vi "Buscador de calor.vi"() -> ()   [LabVIEW 2010]
uses:
  <vilib>/Platform/TimedLoop/XDataNode/XDataNode.xnode
  <vilib>/Platform/TimedLoop/XDataNode/timing_clust.ctl
  <vilib>/Platform/TimedLoop/XDataNode/nitl_modes.ctl
  <vilib>/Platform/TimedLoop/XDataNode/wakeup.ctl
  <vilib>/Instr/_visa.llb/VISA Configure Serial Port (Instr).vi
  <vilib>/Platform/TimedLoop/XDataNode/XDNodeRunTimeDep.lvlib
panel:
  out "Lumenes":dbl(slide) scale=0.0..255.0
  out "String":string
  in  "Ajuste":dbl(slide) scale=0.1..1.0
  in  "Set Lumenes":dbl(slide) scale=50.0..255.0
  in  "Automatico/Manual":bool
  out "Temperatura (ºC) vs tiempo":dynamicdata(graph)
  in  "Intensidad Luminica (%)":dbl(knob) scale=10.0..100.0
  in  "Period                :":i64=1000
  in  "Flow control    :":u16(ring) items=["None"=0, "XON/XOFF"=1, "RTS/CTS"=2, "DTR/DSR"=4]
  in  "Stop bits         :":u16(ring)=10 items=["1.0"=10, "1.5"=15, "2.0"=20]
  in  "Paridad            :":u16(ring) items=["None", "Odd", "Even", "Mark", "Space"]
  in  "Data bits          :":u16=8 min=5 max=8 step=1
  in  "VISA resource : name:":refnum<visa-resource-name>="COM1"
  in  "Baud rate         :":u32=9600
  in  "stop":bool
  out "Read buffer":string
  out "var t":u8
  out "Auto 2":bool
  # "CONTROL INTENSIDAD LUMINICA"
  # "Configuracion Serial"
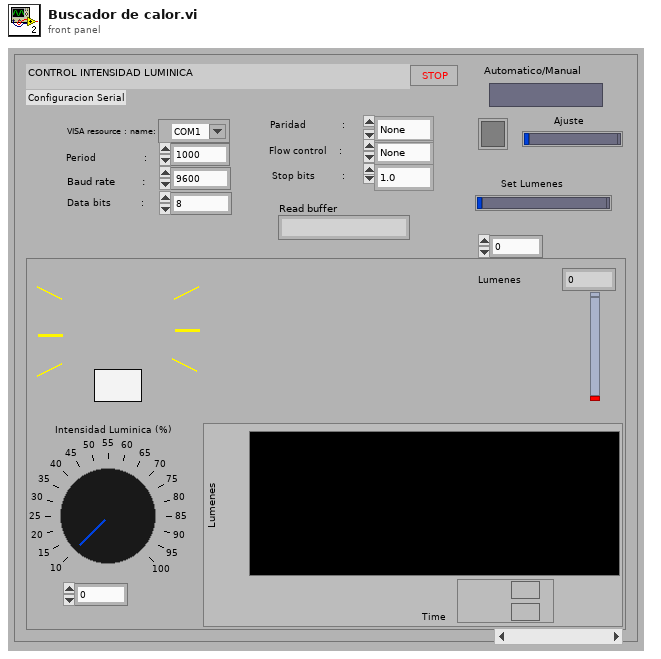
[diagram p1: front panel]
types:
  T1 = typedef "XDNodeRunTimeDep.lvlib/timing_clust.ctl" = cluster{"Expected End [f-1]":u64, "Actual End [f-1]":u64, "Finished Late? [f-1]":bool, "Expected End [i-1]":u64, "Actual End [i-1]":u64, "Finished Late? [i-1]":bool, "Expected Start [i]":u64, "Actual Start [i]":u64, "Expected Start [f]":u64, "Actual Start [f]":u64, "Source Name":string, "Structure Name":string, "Period":i64, "Deadline":i64, "Offset":i64, "Start":i64, "Priority":i32, "Timeout":i32, "Mode":T2, "Wakeup Reason":T3, "Error":errorcluster, "Source Type":string, "Secondary Source Type":string, "Global End Time":u64, "Global Start Time":u64, "Frame Duration":u64, "Iteration Duration":u64, "Assigned CPU":i32, "I/O Scan Engine Mode":u32}
  T2 = typedef "XDNodeRunTimeDep.lvlib/nitl_modes.ctl" = enum32{"No Change", "Process missed periods, maintain original phase", "Discard missed periods, maintain original phase", "Process missed periods, ignore original phase", "Discard missed periods, ignore original phase"}
  T3 = typedef "XDNodeRunTimeDep.lvlib/wakeup.ctl" = enum32{"Normal", "Aborted", "Asynchronous wakeup", "Timing source error", "Timed loop error", "Timeout"}
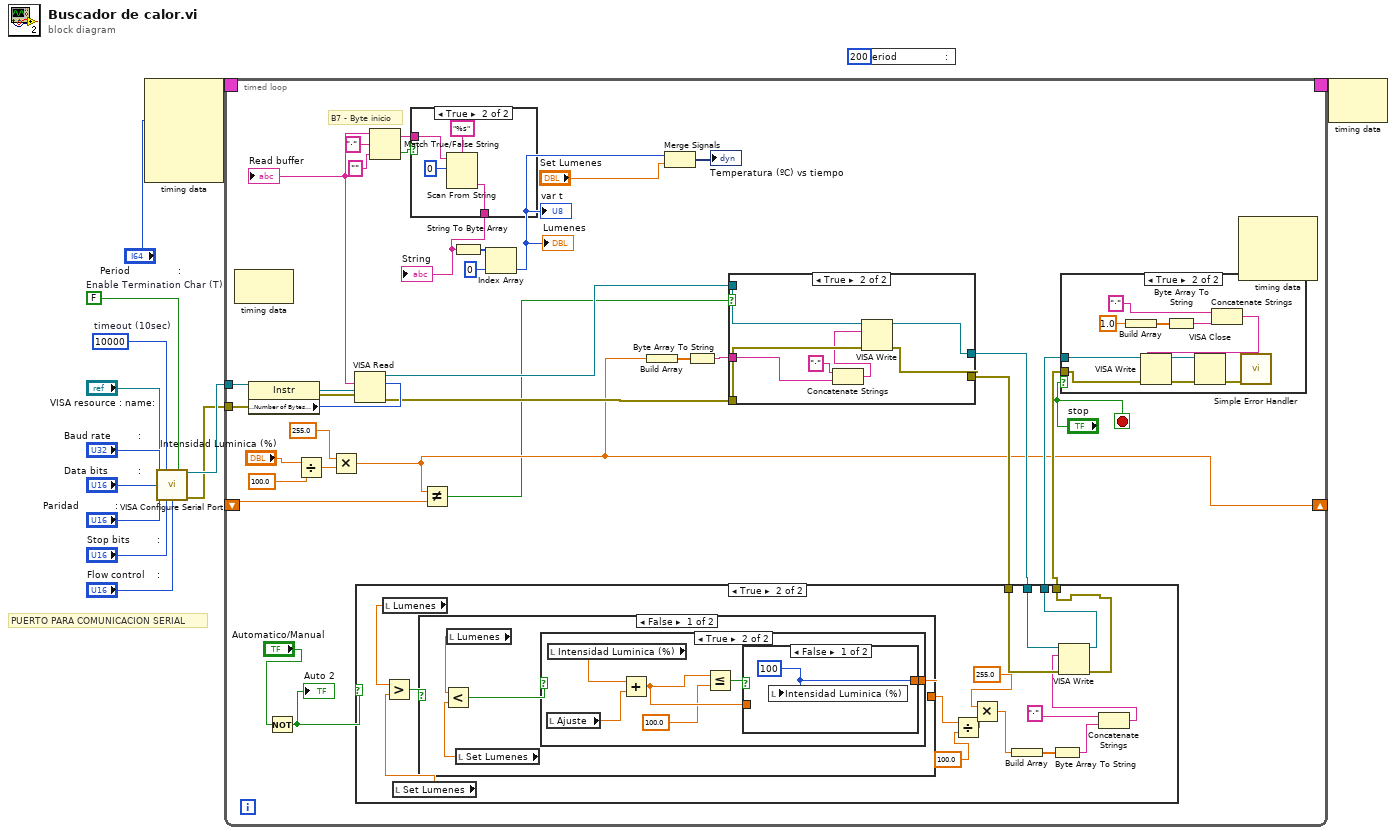
[diagram p0: block diagram]
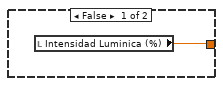
[diagram p3: hidden frame]
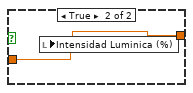
[diagram p4: hidden frame]
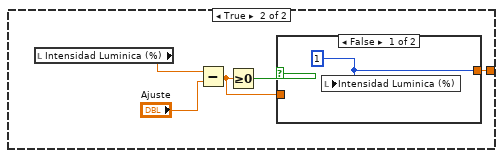
[diagram p5: hidden frame]
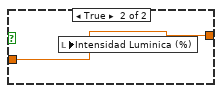
[diagram p6: hidden frame]
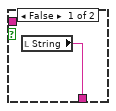
[diagram p8: hidden frame]
diagram:
  w8 = FALSE  # Enable Termination Char (T)
  w9 = u32 10000  # timeout (10sec)
  # "PUERTO PARA COMUNICACION SERIAL"
  n1 = node-c288("Period                :") -> (w14:T1)  [unwired: 4 in]
  n2 = call-poly "VISA Configure Serial Port"("VISA resource name"="VISA resource : name:", "timeout (10sec)"=w9, "Enable Termination\nChar (T)"=w8, "baud rate (9600)"="Baud rate         :", "data bits (8)"="Data bits          :", "parity (0:none)"="Paridad            :", "stop bits (10: 1 bit)"="Stop bits         :", "flow control (0:none)"="Flow control    :") -> ("VISA resource name out"=w4:refnum<visa-resource-name>, "error out"=w3:errorcluster)  [unwired: 6 in]
  n3 = timed-loop {
    timing: w14 -> [_]
    timing-out: [_] -> w13
    tunnel: w4 -> [w41]
    tunnel: w3 -> [w40]
    shift-right: [w16] -> _
    shift-left: _ -> [w36]
    stop <- "stop" stop-if-true
    # "B7 - Byte inicio"
    n4 = node-c288() -> ()  [unwired: 1 in, 1 out]
    n5 = property class="Instr"(reference=w41, error in=w40) -> (reference out=w42:refnum<visa-resource-name>, error out=w37:errorcluster, "Serial Settings:Number of Bytes at Serial Port"=w48:u32)
    n6 = Not(x="Automatico/Manual") -> (.not. x?=w17:bool)
    "Auto 2" <- w17
    n7 = Divide(x="Intensidad Luminica (%)", y=100.0) -> (x/y=w27:dbl)
    n8 = Multiply(x=255.0, y=w27) -> (x*y=w16:dbl)
    n9 = VISA Read(VISA resource name=w42, byte count=w48, error in (no error)=w37) -> (VISA resource name out=w38:refnum<visa-resource-name>, read buffer=w46:string, error out=w34:errorcluster)  [unwired: 1 out]
    "Read buffer" <- w46
    n10 = Match True/False String(2:"" ("false string"), 3:"·" ("true string"), 4:w46) -> (0:w44:bool, 1:w30:string)
    n11 = case shown="True" w44 {
      tunnel: [w96 w98] -> w33
      tunnel: w30 -> [_ w97]
      frame False {
        n12 = local read "String"() -> (w96:string)
      }
      frame True {
        n13 = Scan From String(format string="%s", input string=w97, initial scan location=u32 0) -> (output 1=w98:string)  [unwired: 2 in, 3 out]
      }
    }
    "String" <- w33
    n14 = Not Equal?(x=w16, y=w36) -> (x != y?=w15:bool)
    n15 = String To Byte Array(string=w33) -> (unsigned byte array=w32:u8[])
    n16 = Index Array(array=w32, index=0) -> (element=w22:u8)
    "var t" <- w22
    "Lumenes" <- w22
    n17 = Build Array(w16) -> (w35:dbl[])
    n18 = Merge Signals(w22, "Set Lumenes") -> (→"Temperatura (ºC) vs tiempo":dynamicdata)
    n19 = Byte Array To String(unsigned byte array=w35) -> (string=w39:string)
    n20 = case shown="True" w15 {
      tunnel: w38 -> [w87 w95]
      tunnel: w34 -> [w88 w94]
      tunnel: [w87 w90] -> w20
      tunnel: [w88 w91] -> w21
      tunnel: w39 -> [_ w89]
      frame False {
      }
      frame True {
        n21 = Concatenate Strings("·" ("string"), w89) -> (w92:string)
        n22 = VISA Write(VISA resource name=w95, write buffer=w92, error in (no error)=w94) -> (VISA resource name out=w90:refnum<visa-resource-name>, error out=w91:errorcluster)  [unwired: 1 out]
      }
    }
    n23 = case shown="True" w17 {
      tunnel: w21 -> [w49 w63]
      tunnel: w20 -> [w50 w64]
      tunnel: [w49 w61] -> w19
      tunnel: [w50 w62] -> w18
      frame False {
      }
      frame True {
        n24 = local read "Lumenes"() -> (w66:dbl)
        n25 = local read "Set Lumenes"() -> (w52:dbl)
        n26 = Greater?(x=w66, y=w52) -> (0:w65:bool)
        n27 = case shown="False" w65 {
          tunnel: [w67 w80] -> w55
          frame False {
            n28 = local read "Lumenes"() -> (w70:dbl)
            n29 = local read "Set Lumenes"() -> (w69:dbl)
            n30 = Less?(x=w70, y=w69) -> (x < y?=w68:bool)
            n31 = case shown="True" w68 {
              tunnel: [w71 w73] -> w67
              frame False {
                n32 = local read "Intensidad Luminica (%)"() -> (w71:dbl)
              }
              frame True {
                n33 = local read "Ajuste"() -> (w72:dbl)
                n34 = local read "Intensidad Luminica (%)"() -> (w77:dbl)
                n35 = Add(x=w77, y=w72) -> (x+y=w75:dbl)
                n36 = Less Or Equal?(x=w75, y=100.0) -> (x <= y?=w76:bool)
                n37 = case shown="False" w76 {
                  tunnel: w75 -> [_ w79]
                  tunnel: [w78 w79] -> w73
                  frame False {
                    w78 = u8 100 ("Distancia")
                    n38 = local write "Intensidad Luminica (%)"(w78) -> ()
                  }
                  frame True {
                    n39 = local write "Intensidad Luminica (%)"(w79) -> ()
                  }
                }
              }
            }
          }
          frame True {
            n40 = local read "Intensidad Luminica (%)"() -> (w84:dbl)
            n41 = Subtract(x=w84, y="Ajuste") -> (x-y=w81:dbl)
            n42 = Greater Or Equal To 0?(x=w81) -> (x >= 0?=w82:bool)
            n43 = case shown="False" w82 {
              tunnel: w81 -> [_ w86]
              tunnel: [w85 w86] -> w80
              frame False {
                w85 = u8 1 ("Distancia")
                n44 = local write "Intensidad Luminica (%)"(w85) -> ()
              }
              frame True {
                n45 = local write "Intensidad Luminica (%)"(w86) -> ()
              }
            }
          }
        }
        n46 = Divide(x=w55, y=100.0) -> (x/y=w56:dbl)
        n47 = Multiply(x=255.0, y=w56) -> (x*y=w51:dbl)
        n48 = Build Array(w51) -> (w57:dbl[])
        n49 = Byte Array To String(unsigned byte array=w57) -> (string=w59:string)
        n50 = Concatenate Strings("·" ("string"), w59) -> (w58:string)
        n51 = VISA Write(VISA resource name=w64, write buffer=w58, error in (no error)=w63) -> (VISA resource name out=w62:refnum<visa-resource-name>, error out=w61:errorcluster)  [unwired: 1 out]
      }
    }
    n52 = case shown="True" "stop" {
      tunnel: w19 -> [_ w106]
      tunnel: w18 -> [_ w105]
      frame False {
      }
      frame True {
        n53 = Build Array(1.0 ("element")) -> (w103:dbl[])
        n54 = Byte Array To String(unsigned byte array=w103) -> (string=w102:string)
        n55 = Concatenate Strings("·" ("string"), w102) -> (w107:string)
        n56 = VISA Write(VISA resource name=w105, write buffer=w107, error in (no error)=w106) -> (VISA resource name out=w109:refnum<visa-resource-name>, error out=w108:errorcluster)  [unwired: 1 out]
        n57 = VISA Close(VISA resource name=w109, error in (no error)=w108) -> (error out=w110:errorcluster)
        n58 = call <vilib>:"Simple Error Handler.vi"("error in (no error)"=w110) -> ()  [unwired: 4 in, 5 out]
      }
    }
    n59 = node-c288() -> ()  [unwired: 3 in, 1 out]
  }
  n60 = local write "Period                :"(i64 200 ("Period")) -> ()
  n61 = node-c288(w13) -> ()  [unwired: 1 out]
